vi "ProducerConsumerEvents.vi"() -> ()   [LabVIEW 2019]
doc: "Use this template to build a producer/consumer design pattern with events to produce queue items. Use this design pattern instead of the User Interface Event Handler pattern for user interfaces when you want to execute code asynchronously in response to an event without slowing the user interface responsiveness."
panel:
  out "Action Run":string
  in  "Action 3":bool
  in  "Action 2":bool
  in  "Action 1":bool
  in  "stop":bool
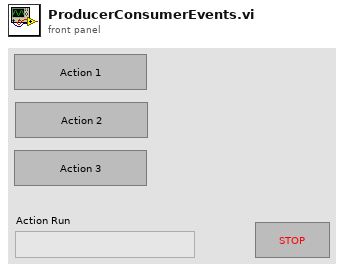
[diagram p1: front panel]
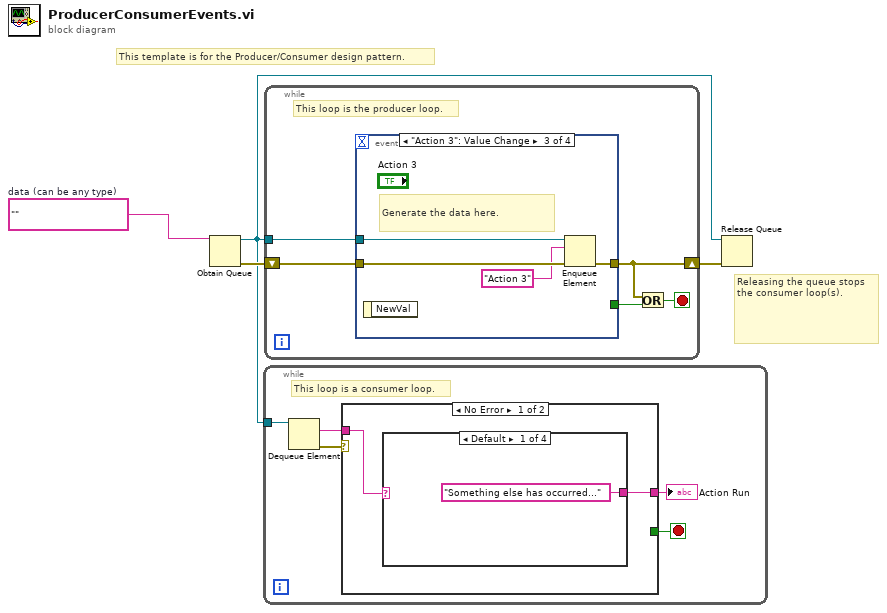
[diagram p0: block diagram]
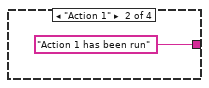
[diagram p2: hidden frame]
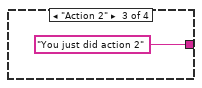
[diagram p3: hidden frame]
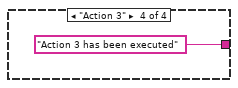
[diagram p4: hidden frame]
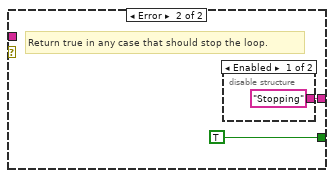
[diagram p5: hidden frame]
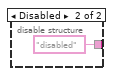
[diagram p6: hidden frame]
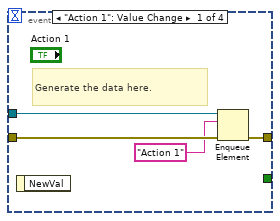
[diagram p7: hidden frame]
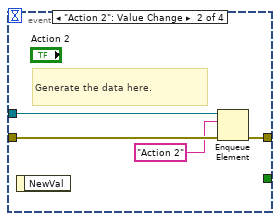
[diagram p8: hidden frame]
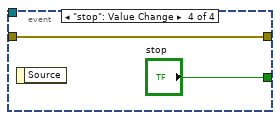
[diagram p9: hidden frame]
diagram:
  w2 = ""  # data (can be any type)
  # "Releasing the queue stops the consumer loop(s)."
  # "This template is for the Producer/Consumer design pattern."
  n1 = Obtain Queue(element data type=w2) -> (queue out=w1:refnum<queue>, error out=w4:errorcluster)  [unwired: 4 in, 1 out]
  n2 = while {
    tunnel: w1 -> [w9]
    stop <- w6 stop-if-true
    # "This loop is a consumer loop."
    n3 = Dequeue Element(queue=w9) -> (element=w7:string, error out=w8:errorcluster)  [unwired: 2 in, 2 out]
    n4 = case shown="No Error" w8 {
      tunnel: w7 -> [w10 _]
      tunnel: [_ TRUE] -> w6
      tunnel: [w11 w16] -> w5
      frame No Error {
        n5 = case shown="Default" w10 {
          tunnel: ["Something else has occurred..." ("Action Run") "Action 1 has been run" ("Action Run") "You just did action 2" ("Action Run") "Action 3 has been executed" ("Action Run")] -> w11
          frame Default {
          }
          frame "Action 1" {
          }
          frame "Action 2" {
          }
          frame "Action 3" {
          }
        }
      }
      frame Error {
        # "Return true in any case that should stop the loop."
        n6 = disable-structure shown="Enabled" {
          disable-tunnel: ["Stopping" ("Action Run") "disabled" ("Action Run")] -> w16
          frame Enabled {
          }
          frame Disabled {
          }
        }
      }
    }
    "Action Run" <- w5
  }
  n7 = while {
    shift-right: [w20] -> w3
    shift-left: w4 -> [w23]
    tunnel: w1 -> [w24]
    stop <- w21 stop-if-true
    # "This loop is the producer loop."
    n8 = event shown="[2] \"Action 3\": Value Change" {
      selector: _ -> [_ _ _ _]
      dyn-events: _ -> [_ _ _ _]
      timeout: _ -> [_ _ _ _]
      tunnel: w24 -> [w28 w32 w36 _]
      tunnel: w23 -> [w27 w31 w35 w37]
      tunnel: [w26 w30 w34 w37] -> w20
      tunnel: [_ _ _ "stop"] -> w22
      event "Action 1": Value Change {
        # "Generate the data here."
        n9 = event-data() -> ()  [unwired: 1 in, 1 out]
        n10 = Enqueue Element(queue=w28, element="Action 1", error in (no error)=w27) -> (error out=w26:errorcluster)  [unwired: 1 in, 2 out]
      }
      event "Action 2": Value Change {
        # "Generate the data here."
        n11 = event-data() -> ()  [unwired: 1 in, 1 out]
        n12 = Enqueue Element(queue=w32, element="Action 2", error in (no error)=w31) -> (error out=w30:errorcluster)  [unwired: 1 in, 2 out]
      }
      event "Action 3": Value Change {
        # "Generate the data here."
        n13 = event-data() -> ()  [unwired: 1 in, 1 out]
        n14 = Enqueue Element(queue=w36, element="Action 3", error in (no error)=w35) -> (error out=w34:errorcluster)  [unwired: 1 in, 2 out]
      }
      event "stop": Value Change {
        n15 = event-data() -> ()  [unwired: 1 in, 1 out]
      }
    }
    n16 = Or(x=w20, y=w22) -> (x .or. y?=w21:bool)
  }
  n17 = Release Queue(queue=w1, error in (no error)=w3) -> ()  [unwired: 1 in, 3 out]
